vi "Get Digital Reader Current Values Queue.vi"(8 "error in (no error)":errorcluster, 10 "Queue of Queue":refnum<queue>, 11 "Digital Reader in":refnum<class "Digital Reader.lvclass">) -> (0 "error out":errorcluster, 3 "Digital Reader out":refnum<class "Digital Reader.lvclass">)   [LabVIEW 2024, in "DAQmx Actor.lvlib" / "Digital Reader.lvclass"]
uses:
  Digital Reader.lvclass
  Digital Reader.lvclass/Digital Reader.ctl
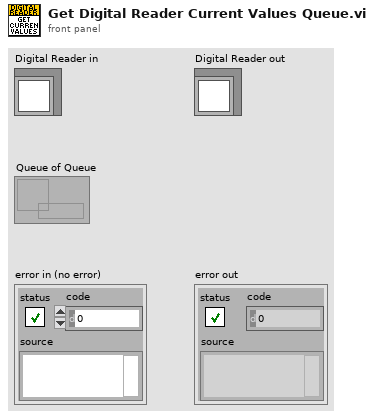
[diagram p1: front panel]
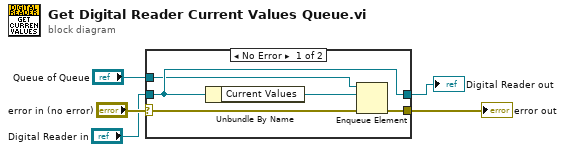
[diagram p0: block diagram]
diagram:
  n1 = case shown="No Error" "error in (no error)" {
    selector: "error in (no error)" -> [w8 w12]
    tunnel: [w7 w12] -> w4
    tunnel: [w10 w11] -> w2
    tunnel: "Digital Reader in" -> [w10 w11]
    tunnel: "Queue of Queue" -> [w9 _]
    frame No Error {
      n2 = Unbundle By Name(w10) -> ("Current Values"=w6:refnum<queue>)
      n3 = Enqueue Element(queue=w9, element=w6, error in (no error)=w8) -> (error out=w7:errorcluster)  [unwired: 1 in, 2 out]
    }
    frame Error {
    }
  }
  "error out" <- w4
  "Digital Reader out" <- w2
